vi "searchVi.vi"(8 "error in (no error)":errorcluster, 10 "regExpr":string, 11 "LibReader in":refnum<class "LibReader.lvclass">) -> (0 "error out":errorcluster, 1 "pathVi":path, 2 "foundVi":bool, 3 "LibReader out":refnum<class "LibReader.lvclass">)   [LabVIEW 2018, in "LibReader.lvclass"]
doc: "Search the vi in lvlib."
uses:
  LibReader.lvclass
  LibReader.lvclass/LibReader.ctl
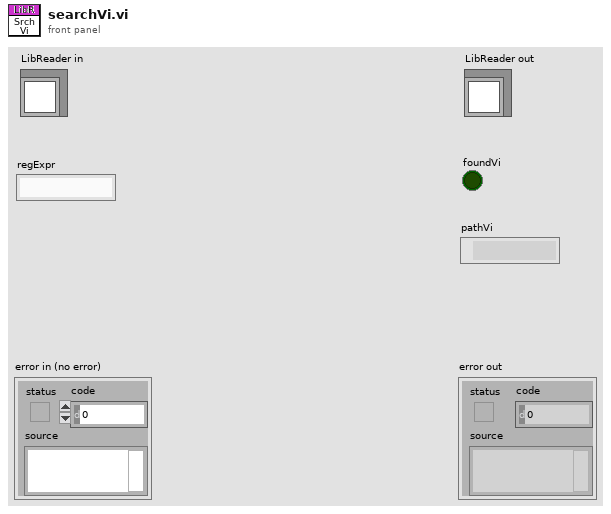
[diagram p1: front panel]
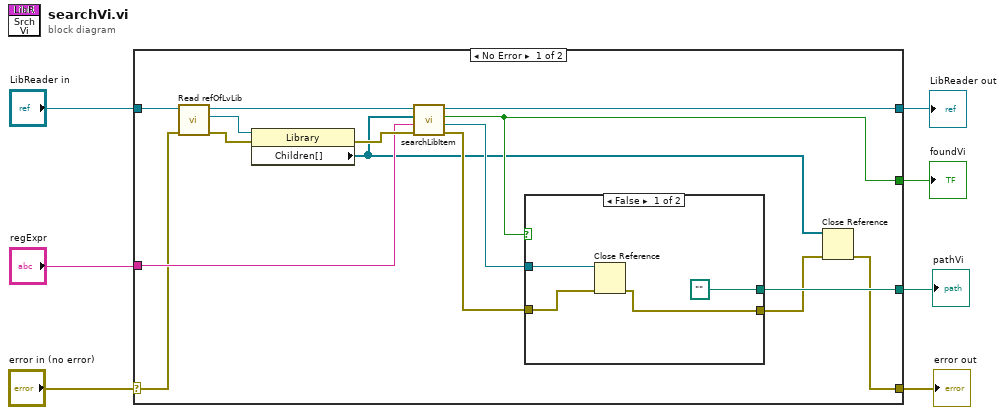
[diagram p0: block diagram]
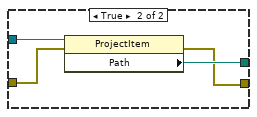
[diagram p2: hidden frame]
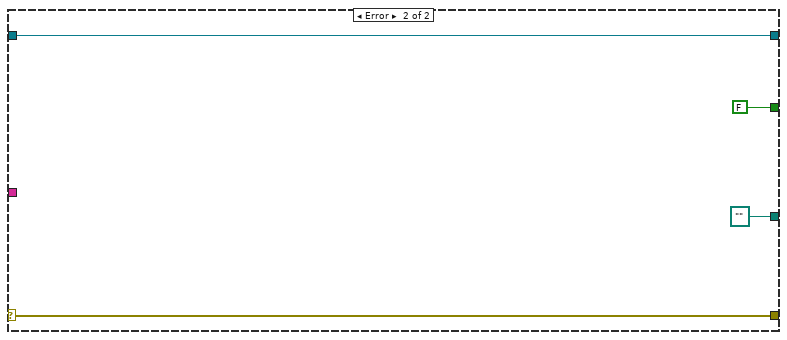
[diagram p3: hidden frame]
diagram:
  n1 = case shown="No Error" "error in (no error)" {
    selector: "error in (no error)" -> [w14 w34]
    tunnel: [w9 w34] -> w6
    tunnel: [w11 w33] -> w2
    tunnel: "LibReader in" -> [w21 w33]
    tunnel: "regExpr" -> [w19 _]
    tunnel: [w18 FALSE] -> w4
    tunnel: [w15 path "" ("Path")] -> w3
    frame No Error {
      n2 = call "Read refOfLvLib.vi"("error in (no error)"=w14, "LibReader in"=w21) -> ("error out"=w13:errorcluster, "refOfLvLib"=w22:refnum<vi>, "LibReader out"=w12:refnum<class "LibReader.lvclass">)  [unwired: 7 in]
      n3 = property class="Library"(reference=w22, error in=w13) -> (error out=w20:errorcluster, "Children[]"=w8:refnum<vi>[])  [unwired: 1 out]
      n4 = call "searchLibItem.vi"("error in (no error)"=w20, "regExpr"=w19, "Owned Items[]"=w8, "LibReader in"=w12) -> ("error out"=w16:errorcluster, "ProjectItem Refnum"=w17:refnum<vi>, "found"=w18:bool, "LibReader out"=w11:refnum<class "LibReader.lvclass">)  [unwired: 4 in]
      n5 = case shown="False" w18 {
        tunnel: w17 -> [w25 w30]
        tunnel: w16 -> [w24 w29]
        tunnel: [path "" ("Path") w28] -> w15
        tunnel: [w23 w27] -> w10
        frame False {
          n6 = Close Reference(reference=w25, error in (no error)=w24) -> (error out=w23:errorcluster)
        }
        frame True {
          n7 = property class="ProjectItem"(reference=w30, error in=w29) -> (error out=w27:errorcluster, "Path"=w28:path)  [unwired: 1 out]
        }
      }
      n8 = Close Reference(reference=w8, error in (no error)=w10) -> (error out=w9:errorcluster)
    }
    frame Error {
    }
  }
  "error out" <- w6
  "LibReader out" <- w2
  "foundVi" <- w4
  "pathVi" <- w3
